vi "SystemController.InitializeImageBuffer.vi"(8 "error in (no error)":errorcluster, 11 "SystemController":refnum<class "SystemController.lvclass">) -> (0 "error out":errorcluster, 3 "SystemController out":refnum<class "SystemController.lvclass">)   [LabVIEW 2017, in "SystemController.lvclass"]
doc: "---------------------------------------------------------------\nJKI State Machine Objects™\nhttp://jki.net/state-machine-objects/\nCopyright (C) 2005-2015, JKI <info@jki.net>\nALL RIGHTS RESERVEDJKI State Machine Objects (SMO) 1.0.0.5\nJKI - JKI\nCopyright (c) 2016, JKI"
uses:
  SystemController.lvclass
  SystemController.lvclass/SystemController.ctl
panel:
  # "For instructions on how to use the JKI State Machine Objects, examples and video tutorials, visit:\nhttp://jki.net/state-machine-objects/\n\nJKI State Machine Objects™\nhttp://jki.net/state-machine-objects/\nCopyright (C) 2005-2015, JKI <info@jki.net>\nALL RIGHTS RESERVED"
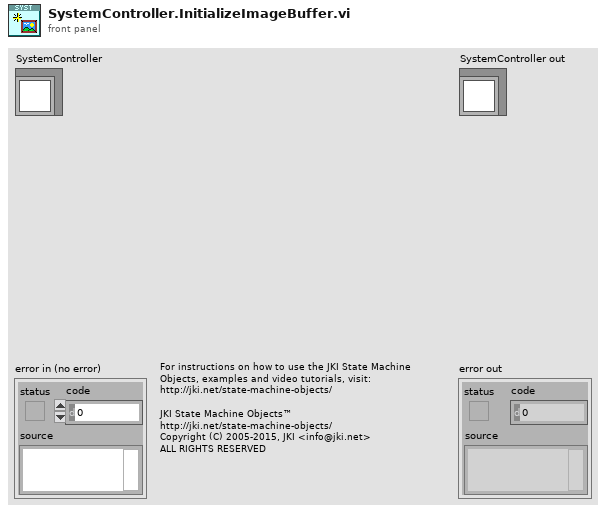
[diagram p1: front panel]
types:
  T1 = typedef "SystemController.lvclass/Configuration--Cluster.ctl" = cluster{"Camera":T2, "Find Eyes":bool, "Acquisition Rate (ms)":i32, "Image Buffer Length":i32}
  T2 = typedef "SystemController.lvclass/CameraConfig--Cluster.ctl" = cluster{"Simulate Camera":bool, "IMAQ Camera":T3, "Simulated Image Folder":path}
  T3 = typedef "Camera_IMAQdx.lvclass/Configuration--Cluster.ctl" = cluster{"Camera Interface Name":string, "Number of Buffers":u32, "Image Name":string, "Image Type":T4}
  T4 = typedef "Image Type" = u32
  T5 = typedef "IMAQ Image.ctl" = refnum<image>
  T6 = typedef "SystemController.lvclass/PrivateData--Ref.ctl" = refnum<data-value>
  T7 = typedef "SystemController.lvclass/PrivateData--Cluster.ctl" = cluster{"Configuration":T1, "Dependencies":T8, "Public Events":T9, "Processed Image Buffer":T5[]}
  T8 = typedef "SystemController.lvclass/Dependencies--Cluster.ctl" = cluster{"Camera":refnum<class "Camera.lvclass">, "ImageFacialDetection":refnum<class "ImageFacialDetection.lvclass">}
  T9 = typedef "SystemController.lvclass/PublicEvents--Cluster.ctl" = cluster{"UIClosed":refnum<user-event>}
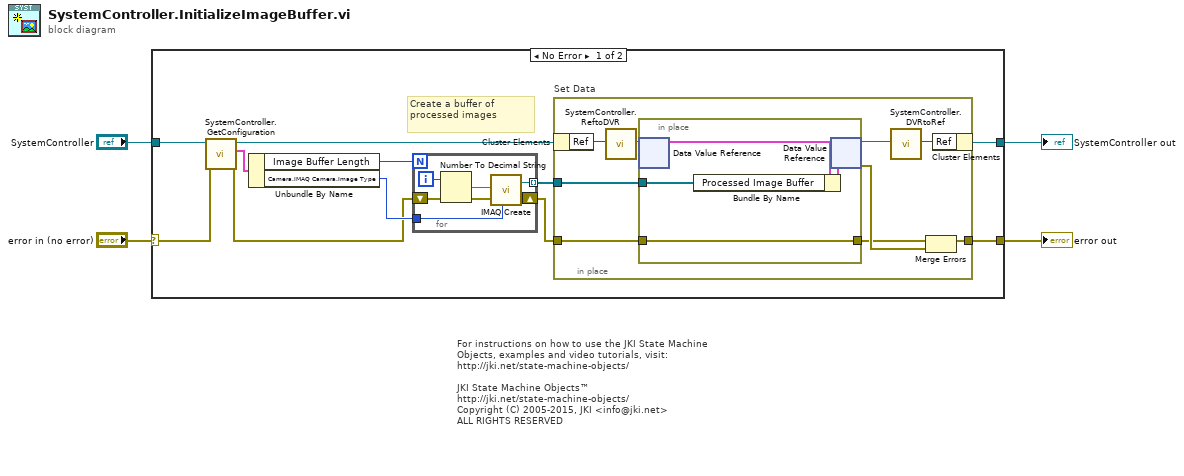
[diagram p0: block diagram]
diagram:
  # "For instructions on how to use the JKI State Machine Objects, examples and video tutorials, visit:\nhttp://jki.net/state-machine-objects/\n\nJKI State Machine Objects™\nhttp://jki.net/state-machine-objects/\nCopyright (C) 2005-2015, JKI <info@jki.net>\nALL RIGHTS RESERVED"
  n1 = case shown="No Error" "error in (no error)" {
    selector: "error in (no error)" -> [w11 w35]
    tunnel: "SystemController" -> [w15 w36]
    tunnel: [w14 w35] -> w3
    tunnel: [w13 w36] -> w2
    frame No Error {
      # "Create a buffer of processed images"
      n2 = call "SystemController.GetConfiguration.vi"("error in (no error)"=w11, "SystemController"=w15) -> ("error out"=w6:errorcluster, "Configuration"=w10:T1, "SystemController out"=w12:refnum<class "SystemController.lvclass">)  [unwired: 7 in]
      n3 = Unbundle By Name(w10) -> ("Image Buffer Length"=w9:i32, "Camera.IMAQ Camera.Image Type"=w7:T4)
      n4 = for {
        N: w9 -> [_]
        tunnel: [w19] -> w8 mode=indexing
        shift-right: [w17] -> w5
        shift-left: w6 -> [w18]
        tunnel: w7 -> [w16]
        i -> [w21]
        n5 = Number To Decimal String(number=w21) -> (decimal integer string=w20:string)  [unwired: 1 in]
        n6 = call "IMAQ Create"("Image Name"=w20, "Image Type"=w16, "error in (no error)"=w18) -> ("New Image"=w19:T5, "error out"=w17:errorcluster)  [unwired: 2 in]
      }
      n7 = in-place "Set Data" {
        in-place-border: w5 -> [w30]
        in-place-border: [w27] -> w14
        in-place-border: w8 -> [w22]
        n8 = in-place-cluster #1(w12) -> ("Ref"=w26:u32)
        n9 = call "SystemController.ReftoDVR.vi"("Ref"=w26) -> ("Ref"=w25:T6)  [unwired: 10 in]
        n10 = in-place {
          in-place-border: w30 -> [w33]
          in-place-border: [w33] -> w28
          in-place-border: w22 -> [w31]
          n11 = in-place-dvr #2(w25) -> (w34:T7)  [unwired: 1 out]
          n12 = Bundle By Name(cluster=w34, "Processed Image Buffer"=w31) -> (w32:T7)
          n13 = in-place-dvr #2(w32) -> (w24:T6, w29:errorcluster)
        }
        n14 = call "SystemController.DVRtoRef.vi"("Ref"=w24) -> ("Ref"=w23:u32)  [unwired: 10 in]
        n15 = Merge Errors(w28, w29) -> (w27:errorcluster)
        n16 = in-place-cluster #1("Ref"=w23) -> (w13:refnum<class "SystemController.lvclass">)
      }
    }
    frame Error {
    }
  }
  "error out" <- w3
  "SystemController out" <- w2
